vi "PCO_GetCoolingSetpoints.vi"(8 "error in (no error)":errorcluster {"code" format="%x"}, 9 "wNumSetPoints":u16, 10 "wBlockID":u16, 11 "ph":u64) -> (0 "error out":errorcluster {"code" format="%x"}, 1 "wNumSetPoints out":u16, 2 "ErrorMessage":i32 format="%x", 3 "ph out":u64, 5 "sCoolSetpoints":i16[](array[numeric]))   [LabVIEW 2019, in "SDK.lvlib" / "ImageSensor.lvlib"]
doc: "<b>Description:</b>\nThis function gets the cooling setpoints of the camera. This is used when no minimum or maximum range is available.\n\n<b>Supported camera type:</b>\nAll cameras\n\n<b>Descriptor dependency:</b>\ndwGeneralCapsDESC1: COOLING_SETPOINTS"
uses:
  ImageSensor.lvlib
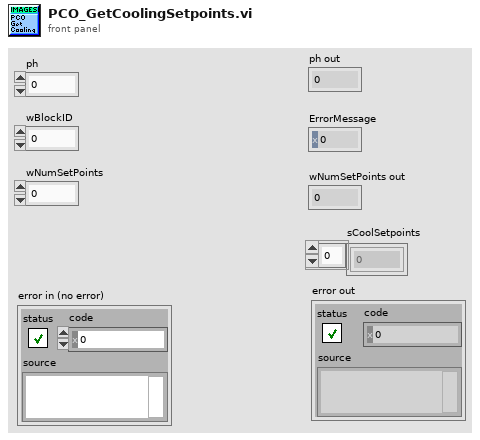
[diagram p1: front panel]
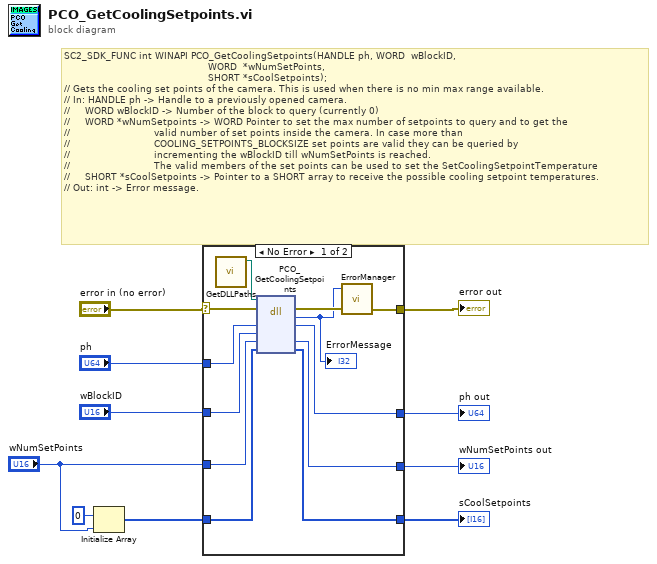
[diagram p0: block diagram]
diagram:
  # "SC2_SDK_FUNC int WINAPI PCO_GetCoolingSetpoints(HANDLE ph, WORD  wBlockID,\n                                                WORD  *wNumSetPoints,\n                                                SHORT *sCoolSetpoints);\n// Gets the cooling set points of the camera. This is used when there is no min max range available.\n// In: HANDLE ph -> Handle to a previously opened camera.\n//     WORD wBlockID -> Number of the block to query (currently 0)\n//     WORD *wNumSetpoints -> WORD Pointer to set the max number of setpoints to query and to get the\n//                            valid number of set points inside the camera. In case more than\n//                            COOLING_SETPOINTS_BLOCKSIZE set points are valid they can be queried by\n//                            incrementing the wBlockID till wNumSetPoints is reached.\n//                            The valid members of the set points can be used to set the SetCoolingSetpointTemperature\n//     SHORT *sCoolSetpoints -> Pointer to a SHORT array to receive the possible cooling setpoint temperatures.\n// Out: int -> Error message."
  n1 = Initialize Array(i16 0 ("element"), "wNumSetPoints") -> (w2:i16[])
  n2 = case shown="No Error" "error in (no error)" {
    selector: "error in (no error)" -> [w12 w26]
    tunnel: "ph" -> [w22 w25]
    tunnel: [w21 w25] -> w9
    tunnel: "wBlockID" -> [w20 _]
    tunnel: "wNumSetPoints" -> [w19 w24]
    tunnel: [w18 w24] -> w7
    tunnel: w2 -> [w17 w23]
    tunnel: [w16 w23] -> w6
    tunnel: [w14 w26] -> w5
    frame No Error {
      n3 = call "GetDLLPaths.vi"() -> ("SC2_Cam_Path"=w11:path)  [unwired: 8 in, 3 out]
      n4 = dll-call lib="?" fn="PCO_GetCoolingSetpoints"(path in=w11, error in=w12, "ph"=w22, "wBlockID"=w20, "wNumSetPoints"=w19, "sCoolSetpoints"=w17) -> (error out=w15:errorcluster, "return type"=w13:i32, "ph"=w21:u64, "wNumSetPoints"=w18:u16, "sCoolSetpoints"=w16:i16[])  [unwired: 2 in, 1 out]
      "ErrorMessage" <- w13
      n5 = call "ErrorManager.vi"("error in (no error)"=w15, "error code"=w13) -> ("error out"=w14:errorcluster)  [unwired: 2 in, 1 out]
    }
    frame Error {
    }
  }
  "ph out" <- w9
  "wNumSetPoints out" <- w7
  "sCoolSetpoints" <- w6
  "error out" <- w5
